vi "YKMW100 Receive String-clear buff.vi"(0 "VISA session":refnum<visa-resource-name>="MW100", 9 "Timeout (25000)":u32=100, 11 "error in (no error)":errorcluster, 13 "Source (\"\")":string) -> (4 "dup VISA session":refnum<visa-resource-name>, 8 "Read Buffer":string, 15 "error out":errorcluster)   [LabVIEW 2020]
doc: "This VI receives ASCII code string which ends with terminator \"CRLF\" from the instrument. \nThis VI returns read buffer except CRLF."
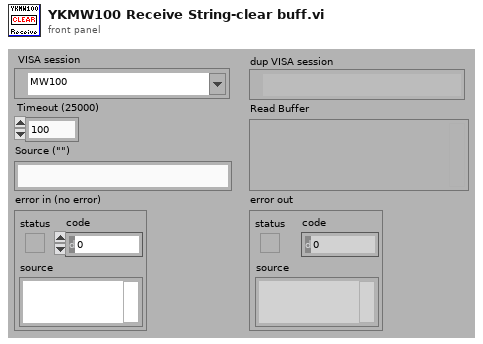
[diagram p1: front panel]
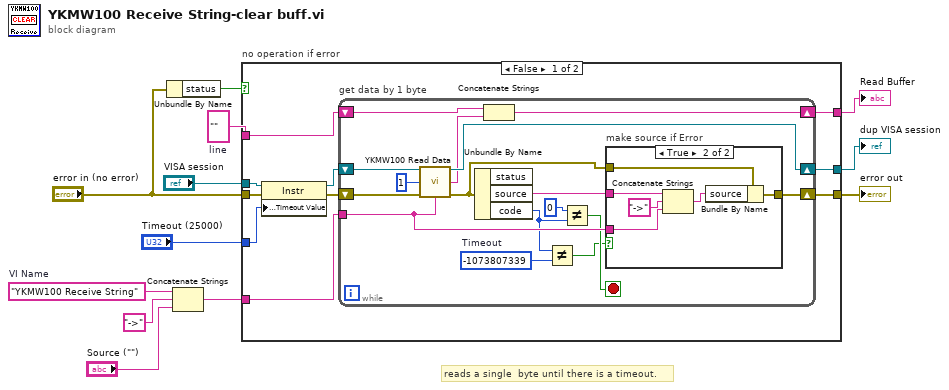
[diagram p0: block diagram]
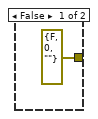
[diagram p2: hidden frame]
diagram:
  w5 = "YKMW100 Receive String"  # VI Name
  w8 = ""  # line
  # "reads a single  byte until there is a timeout."
  n1 = Unbundle By Name("error in (no error)") -> ("status"=w11:bool)
  n2 = Concatenate Strings(w5, "->", "Source (\"\")") -> (w3:string)
  n3 = case "no operation if error" shown="False" w11 {
    tunnel: "VISA session" -> [w15 w48]
    tunnel: [w22 w48] -> w9
    tunnel: [w18 w47] -> w2
    tunnel: "error in (no error)" -> [w17 w47]
    tunnel: w3 -> [w20 _]
    tunnel: [w19 w46] -> w10
    tunnel: w8 -> [w21 w46]
    tunnel: "Timeout (25000)" -> [w13 _]
    frame False {
      n4 = property class="Instr"(reference=w15, error in=w17, "General Settings:Timeout Value"=w13) -> (reference out=w14:refnum<visa-resource-name>, error out=w16:errorcluster)
      n5 = while "get data by 1 byte" {
        shift-left: w16 -> [w34]
        shift-right: [w36] -> w18
        tunnel: w20 -> [w30]
        shift-left: w21 -> [w38]
        shift-right: [w28] -> w19
        shift-right: [w33] -> w22
        shift-left: w14 -> [w35]
        stop <- w24 stop-if-true
        w27 = -1073807339  # Timeout
        n6 = call "YKMW100 Read Data.vi"("VISA session"=w35, "Byte (0)"=1, "error in (no error)"=w34, "Source (\"\")"=w30) -> ("dup VISA session"=w33:refnum<visa-resource-name>, "Read Buffer"=w29:string, "error out"=w32:errorcluster)  [unwired: 9 in]
        n7 = Unbundle By Name(w32) -> ("source"=w37:string, "code"=w26:i32)  [unwired: 1 out]
        n8 = Concatenate Strings(w38, w29) -> (w28:string)
        n9 = Not Equal?(x=w26, y=w27) -> (x != y?=w23:bool)
        n10 = Not Equal?(x=0, y=w26) -> (x != y?=w24:bool)
        n11 = case "make source if Error" shown="True" w23 {
          tunnel: w32 -> [_ w45]
          tunnel: [errorcluster {"status"=FALSE, "code"=0, "source"=""} ("error out") w44] -> w36
          tunnel: w37 -> [_ w42]
          tunnel: w30 -> [_ w40]
          frame False {
          }
          frame True {
            n12 = Concatenate Strings(w42, "->", w40) -> (w41:string)
            n13 = Bundle By Name(cluster=w45, "source"=w41) -> (w44:errorcluster)
          }
        }
      }
    }
    frame True {
    }
  }
  "error out" <- w2
  "dup VISA session" <- w9
  "Read Buffer" <- w10
